vi "GetPluginName.vi"(8 "error in (no error)":errorcluster, 11 "config":string) -> (0 "error out":errorcluster, 2 "Plugin":string, 3 "config(out)":string)   [LabVIEW 2015, in "Serializer.lvlib"]
uses:
  Serializer.lvlib
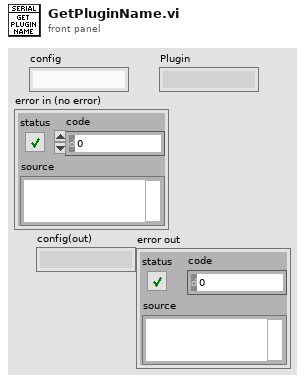
[diagram p1: front panel]
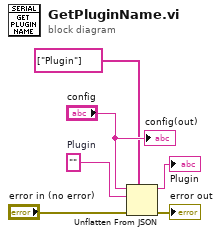
[diagram p0: block diagram]
diagram:
  w4 = ""  # Plugin
  n1 = Unflatten From JSON(path=string[] ["Plugin"], JSON string="config", type and defaults=w4, error in (no error)="error in (no error)") -> (value=→"Plugin":string, error out=→"error out":errorcluster)  [unwired: 3 in]
  "config(out)" <- "config"
